vi "Read I2C Slave Address (0).vi"(8 "error in (no error)":errorcluster, 11 "LINX I2C in":refnum<class "LINX I2C.lvclass">) -> (0 "error out":errorcluster, 2 "I2C Slave Address (0)":u8=64 format="%.0x", 3 "LINX I2C out":refnum<class "LINX I2C.lvclass">)   [LabVIEW 2020, in "LINX I2C.lvclass"]
uses:
  LINX I2C.lvclass
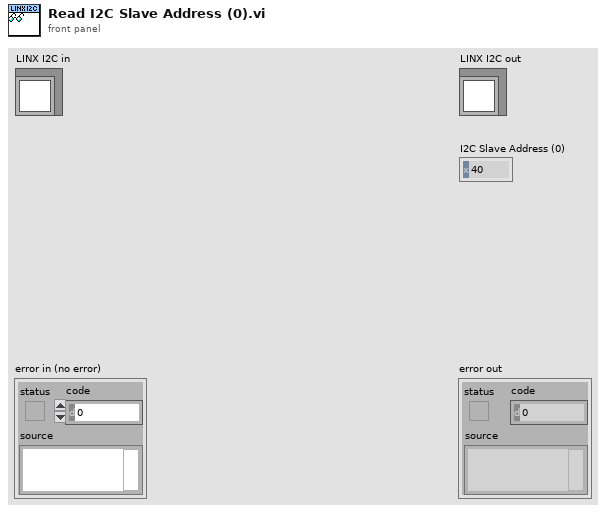
[diagram p1: front panel]
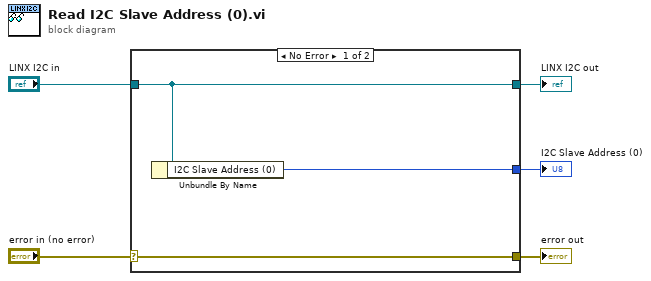
[diagram p0: block diagram]
diagram:
  n1 = case shown="No Error" "error in (no error)" {
    selector: "error in (no error)" -> [w8 w9]
    tunnel: [w8 w9] -> w4
    tunnel: [w7 w10] -> w2
    tunnel: "LINX I2C in" -> [w7 w10]
    tunnel: [w6 _] -> w1
    frame No Error {
      n2 = Unbundle By Name(w7) -> ("I2C Slave Address (0)"=w6:u8)
    }
    frame Error {
    }
  }
  "error out" <- w4
  "LINX I2C out" <- w2
  "I2C Slave Address (0)" <- w1
